vi "classes.vi"(0 "MyAppFactory":refnum<class "MyAppFactory.lvclass">, 1 "className":string, 5 "error in (no error)":errorcluster) -> (14 "MyAppFactory dup":refnum<class "MyAppFactory.lvclass">, 16 "Object":refnum<class>, 19 "error out":errorcluster)   [LabVIEW 2012, in "MyApp.lvlib" / "MyAppFactory.lvclass"]
doc: "This dynamaic dispatch VI contains constant objects of all classes that can be produced by HGF_Factory.\nClass has to be defined by name. \n\nOptionally, you can also specifiy a Class Path String instead, but you have to make sure that all dependencies are available.\n\nChild classes have to override it to define additional classes."
uses:
  MyAppFactory.lvclass
  MyApp.lvclass
  MyAppConfig/MyAppConfig.lvclass
  HGF_LVC/HGF_BaseClasses/HGF_Factory/HGF_Factory.lvclass
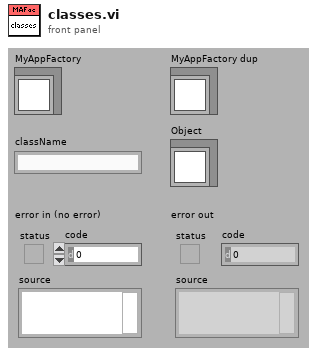
[diagram p1: front panel]
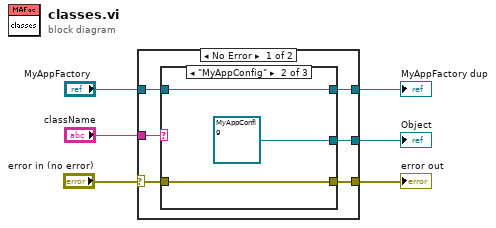
[diagram p0: block diagram]
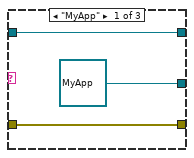
[diagram p2: hidden frame]
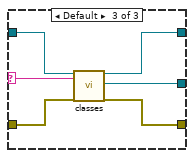
[diagram p3: hidden frame]
diagram:
  n1 = case shown="No Error" "error in (no error)" {
    selector: "error in (no error)" -> [w8 w25]
    tunnel: "MyAppFactory" -> [w12 w26]
    tunnel: "className" -> [w7 _]
    tunnel: [w11 w26] -> w4
    tunnel: [w10 _] -> w3
    tunnel: [w9 w25] -> w2
    frame No Error {
      n2 = case shown="\"MyAppConfig\"" w7 {
        selector: w7 -> [_ _ w19]
        tunnel: w12 -> [w15 w18 w24]
        tunnel: [w15 w18 w23] -> w11
        tunnel: [refnum<class "MyApp.lvclass"> refnum ("MyApp.lvlib:MyApp.lvclass") refnum<class "MyAppConfig.lvclass"> refnum ("MyApp.lvlib:MyAppConfig.lvclass") w22] -> w10
        tunnel: [w14 w17 w21] -> w9
        tunnel: w8 -> [w14 w17 w20]
        frame "MyApp" {
        }
        frame "MyAppConfig" {
        }
        frame Default {
          n3 = call-parent "classes.vi"("HGF_Factory"=w24, "className"=w19, "error in (no error)"=w20) -> ("HGF_Factory dup"=w23:refnum<class "MyAppFactory.lvclass">, "Object"=w22:refnum<class>, "error out"=w21:errorcluster)  [unwired: 14 in]
        }
      }
    }
    frame Error {
    }
  }
  "error out" <- w2
  "MyAppFactory dup" <- w4
  "Object" <- w3
